vi "Read Analogue.vi"(8 "error in (no error)":errorcluster, 11 "Sim Scope in":refnum<class "Sim Scope.lvclass">) -> (0 "error out":errorcluster, 2 "Waveforms":waveform(dbl)[](array[waveform]), 3 "Sim Scope out":refnum<class "Sim Scope.lvclass">)   [LabVIEW 2025, in "Scope.lvlib" / "Sim Scope.lvclass"]
uses:
  Sim Scope.lvclass
  C:/Users/Public/Documents/Sandia National Labs/TSS Plugin/Abstract Engine.lvlibp/Abstract Instrument/Abstract Instrument.lvclass
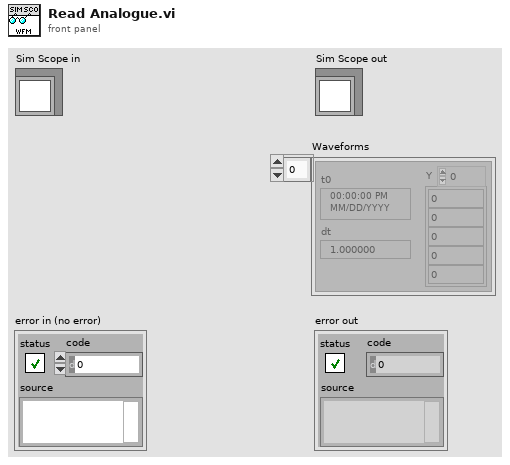
[diagram p1: front panel]
types:
  T1 = typedef "Abstract Engine.lvlibp/Abstract Instrument.lvclass/Channel.ctl" = cluster{"Alias":string, "DataType":enum16{"Anaolg Input", "Waveform"}, "Unit":enum16{"---", "V", "A", "Ohm", "Hz", "uF", "degC", "deg"}, "Upper limit":dbl, "Lower limit":dbl, "Measurement":variant}
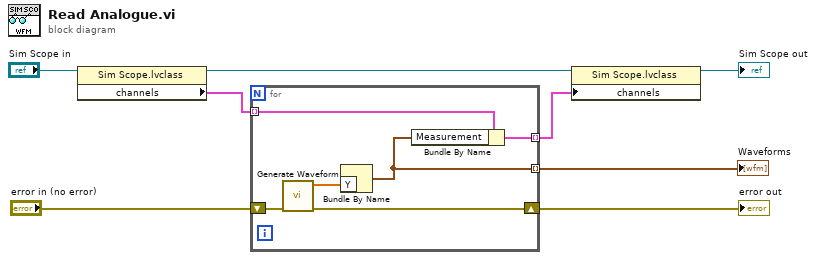
[diagram p0: block diagram]
diagram:
  n1 = property class="Sim Scope.lvclass"(reference="Sim Scope in") -> (reference out=w4:refnum<class "Sim Scope.lvclass">, "channels"=w3:T1[])  [unwired: 1 in, 1 out]
  n2 = for {
    shift-right: [w13] -> w7
    shift-left: "error in (no error)" -> [w14]
    tunnel: w3 -> [w10] mode=indexing
    tunnel: [w11] -> w2 mode=indexing
    tunnel: [w9] -> w1 mode=indexing
    n3 = call "Generate Waveform.vi"("error in (no error)"=w14) -> ("error out"=w13:errorcluster, "Data"=w12:dbl[])  [unwired: 9 in]
    n4 = Bundle By Name("Y"=w12) -> (w9:waveform(dbl))  [unwired: 1 in]
    n5 = Bundle By Name(cluster=w10, "Measurement"=w9) -> (w11:T1)
  }
  "error out" <- w7
  "Waveforms" <- w1
  n6 = property class="Sim Scope.lvclass"(reference=w4, "channels"=w2) -> (reference out=→"Sim Scope out":refnum<class "Sim Scope.lvclass">)  [unwired: 1 in, 1 out]
